vi "FillImagesEnum.vi"() -> ()   [LabVIEW 2015, in "TronviewPresentation.lvlib"]
uses:
  TronviewPresentation.lvlib
  Images.ctl
panel:
  in  "Images folder":path
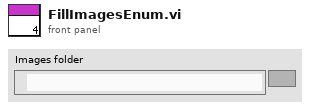
[diagram p1: front panel]
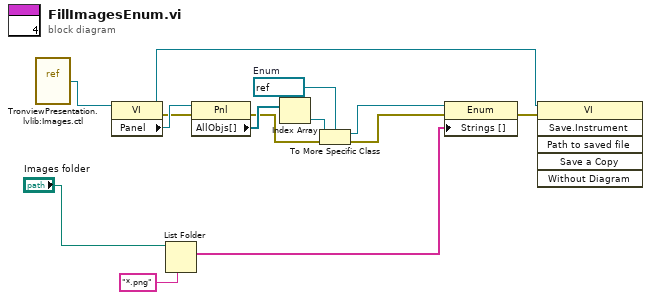
[diagram p0: block diagram]
diagram:
  w10 = refnum<vi> refnum  # Enum
  n1 = vi-ref "TronviewPresentation.lvlib:Images.ctl"() -> (w14:refnum<vi>)
  n2 = property class="VI"(reference=w14) -> (reference out=w1:refnum<vi>, error out=w8:errorcluster, "Panel"=w13:refnum<vi>)  [unwired: 1 in]
  n3 = List Folder(path="Images folder", pattern="*.png") -> (filenames=w3:string[])  [unwired: 2 in, 3 out]
  n4 = property class="Pnl"(reference=w13, error in=w8) -> (error out=w7:errorcluster, "AllObjs[]"=w12:refnum<vi>[])  [unwired: 1 out]
  n5 = Index Array(array=w12) -> (element=w11:refnum<vi>)  [unwired: 1 in]
  n6 = To More Specific Class(target class=w10, reference=w11, error in=w7) -> (specific class reference=w9:refnum<vi>, error out=w6:errorcluster)
  n7 = property class="Enum"(reference=w9, error in=w6, "Strings []"=w3) -> (error out=w2:errorcluster)  [unwired: 1 out]
  n8 = invoke class="VI" method="Save.Instrument"(reference=w1, error in=w2) -> ()  [unwired: 4 in, 6 out]
